vi "Configuration Keys.vi"(8 "error in":errorcluster, 11 "SwitchMatrix in":refnum<class "SwitchMatrix.lvclass">) -> (0 "error out":errorcluster, 2 "Required Keys":string[](array[string]), 3 "SwitchMatrix out":refnum<class "SwitchMatrix.lvclass">)   [LabVIEW 2019, in "SwitchMatrix.lvlib" / "SwitchMatrix.lvclass"]
doc: "Configuration Keys is a dynamic dispatch VI that reads a full inheritance chain's required key list.\n\nThis means each instrument must override this vi, and call the parent method . The end result is a comprehensive list of required keys that must be present in an instrument's config.ini file to correctly function."
uses:
  Library/SwitchMatrix.lvclass
  Custom Controls/Configuration Keys.ctl
  builds/Instruments/Instruments.lvlibp/Library/Instruments.lvclass
panel:
  in  "Configuration Keys":T1
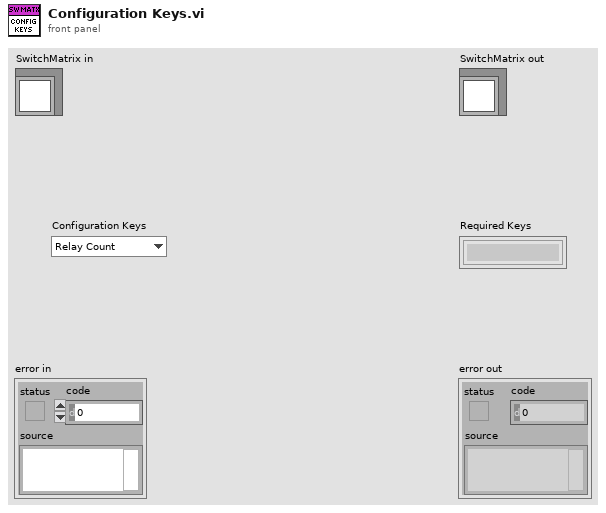
[diagram p1: front panel]
types:
  T1 = typedef "SwitchMatrix.lvlib/SwitchMatrix.lvclass/Configuration Keys.ctl" = enum16{"Relay Count", "Topology"}
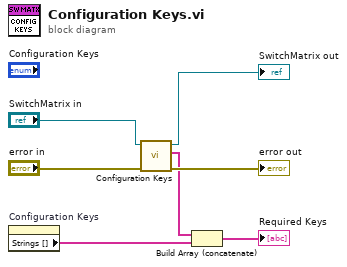
[diagram p0: block diagram]
diagram:
  n1 = property on="Configuration Keys" class="Enum (strict)"() -> ("Strings []"=w3:string[])  [unwired: 2 in, 2 out]
  n2 = call-parent "Configuration Keys.vi"("error in"="error in", "Instruments in"="SwitchMatrix in") -> ("error out"=→"error out":errorcluster, "Required Keys"=w1:string[], "Instruments out"=→"SwitchMatrix out":refnum<class "SwitchMatrix.lvclass">)  [unwired: 7 in]
  n3 = Build Array (concatenate)(w1, w3) -> (→"Required Keys":string[])
